vi "OP30 Verify Station.vi"(2 "Report":i32(listbox), 8 "error in (no error)":errorcluster, 11 "Ref in":T1={"MS SQL Connection"=refnum, "UDL File"=path "", "Time"="", "DCODE"="", "WIP+1"=0, "MC No?"=0, "POKAYOKE?"=FALSE, "Expected Result"="", "Result [Status]"="", "Clock"=0.0, "RFID"="", "WIP Queue"=refnum, "TS Parameter"={"ProfitCenterCode"="", "LineCode"="", "WorkOrderNumber"="", "Model"="", "Model_with_Prefix"="", "VendorCode"="", "SetParameterDateCode"="", "PokaYoke"=0, "Target"=1, "Live_DateCode"="", "CustomerPartNumber"="", "Hand"="", "sBarcode"=FALSE, "FCA"=0, "Ent_Stamp"=timestamp(0 s since 1904-01-01), "STS_CD"=0.0}, "Data_Queue"=[], "RFID Serial No."=""} {"TS Parameter"."FCA" format="%01d"; "TS Parameter"."Target" min=1 max=100000; "TS Parameter"."PokaYoke" min=0 max=1}) -> (0 "error out":errorcluster, 1 "subarray":string[](array[string]), 3 "Ref in 2":T1={"MS SQL Connection"=refnum, "UDL File"=path "", "Time"="", "DCODE"="", "WIP+1"=0, "MC No?"=0, "POKAYOKE?"=FALSE, "Expected Result"="", "Result [Status]"="", "Clock"=0.0, "RFID"="", "WIP Queue"=refnum, "TS Parameter"={"ProfitCenterCode"="", "LineCode"="", "WorkOrderNumber"="", "Model"="", "Model_with_Prefix"="", "VendorCode"="", "SetParameterDateCode"="", "PokaYoke"=0, "Target"=1, "Live_DateCode"="", "CustomerPartNumber"="", "Hand"="", "sBarcode"=FALSE, "FCA"=0, "Ent_Stamp"=timestamp(0 s since 1904-01-01), "STS_CD"=0.0}, "Data_Queue"=[], "RFID Serial No."=""} {"TS Parameter"."FCA" format="%01d"; "TS Parameter"."Target" min=1 max=100000; "TS Parameter"."PokaYoke" min=0 max=1}, 4 "Ack 2":bool)   [LabVIEW 2020]
uses:
  Controls/FV_Status.ctl
  Controls/TD SQL.ctl
  <vilib>/addons/database/Connection.llb/Conn ObjectReference.ctl
  Controls/WIP_State.ctl
  Controls/TS_Parameter.ctl
  <vilib>/Utility/miscctls.llb/LVRowAndColumnUnsignedTypeDef.ctl
  MS SQL/MS_Global.vi
  <vilib>/addons/database/_DB Variant To Data/Database Variant To Data.xnode
  <vilib>/addons/database/NI_Database_API.lvlib
panel:
  in  "Abort":bool
  out "Numeric":i32
  out "x != y?":bool
  in  "RFID_OPC":string="0029032640C1845Ag000001"
  in  "Ack":bool
  out "Over all Status":T4 caption="Data Validation"
  in  "Reason":string
  in  "RFID":string="0029032640C1845Ag000001"
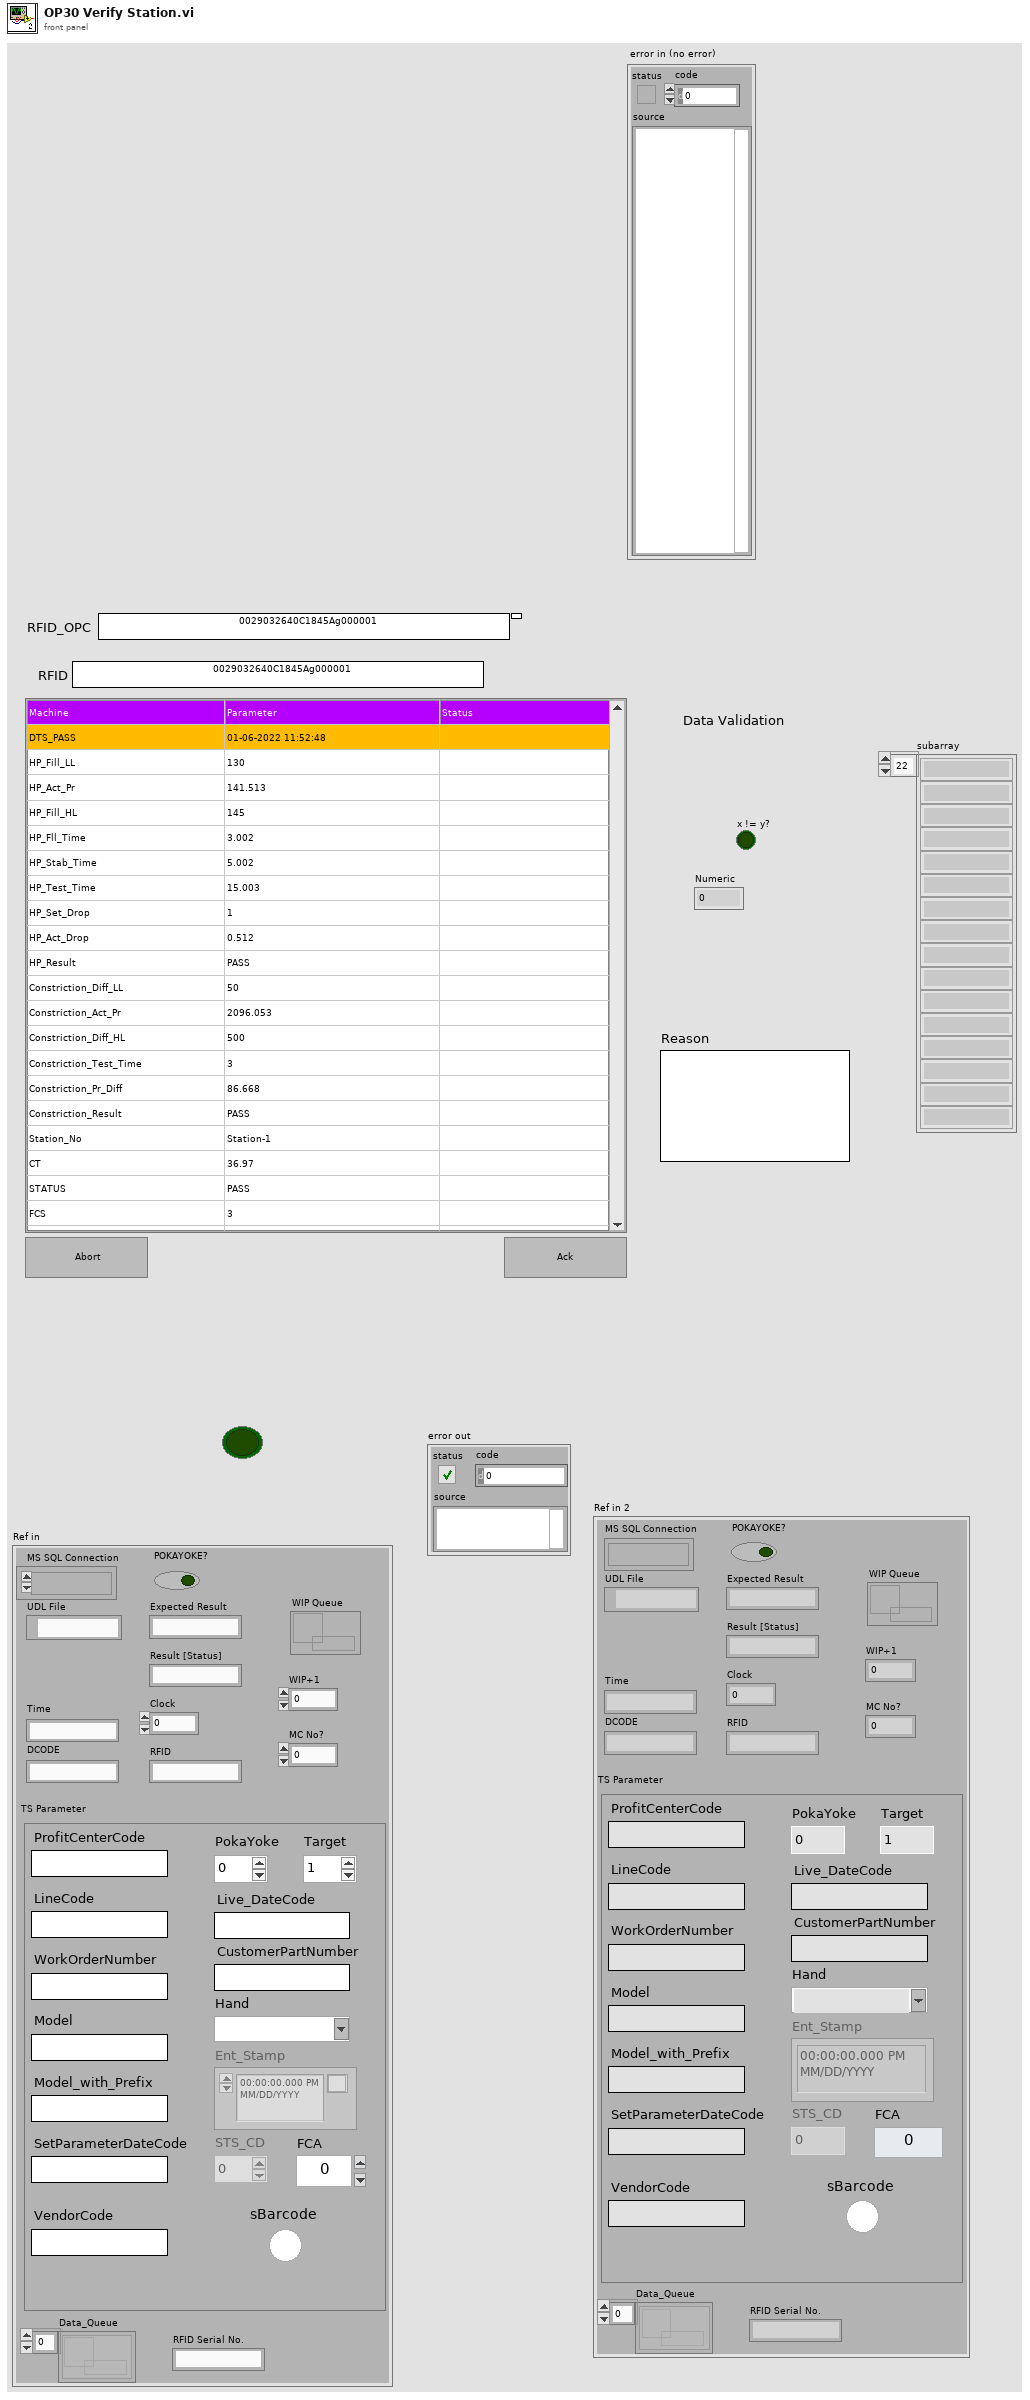
[diagram p1: front panel]
types:
  T1 = typedef "TD SQL.ctl" = cluster{"MS SQL Connection":T2, "UDL File":path, "Time":string, "DCODE":string, "WIP+1":i64, "MC No?":i32, "POKAYOKE?":bool, "Expected Result":string, "Result [Status]":string, "Clock":dbl, "RFID":string, "WIP Queue":refnum<queue>, "TS Parameter":T3, "Data_Queue":refnum<queue>[], "RFID Serial No.":string}
  T2 = typedef "NI_Database_API.lvlib/Conn ObjectReference.ctl" = refnum<k1>
  T3 = typedef "TS_Parameter.ctl" = cluster{"ProfitCenterCode":string, "LineCode":string, "WorkOrderNumber":string, "Model":string, "Model_with_Prefix":string, "VendorCode":string, "SetParameterDateCode":string, "PokaYoke":i32, "Target":i32, "Live_DateCode":string, "CustomerPartNumber":string, "Hand":string, "sBarcode":bool, "FCA":i32, "Ent_Stamp":timestamp, "STS_CD":dbl}
  T4 = typedef "FV_Status.ctl" = u16
  T5 = typedef "LVRowAndColumnUnsignedTypeDef.ctl" = cluster{"Row":u32, "Column":u32}
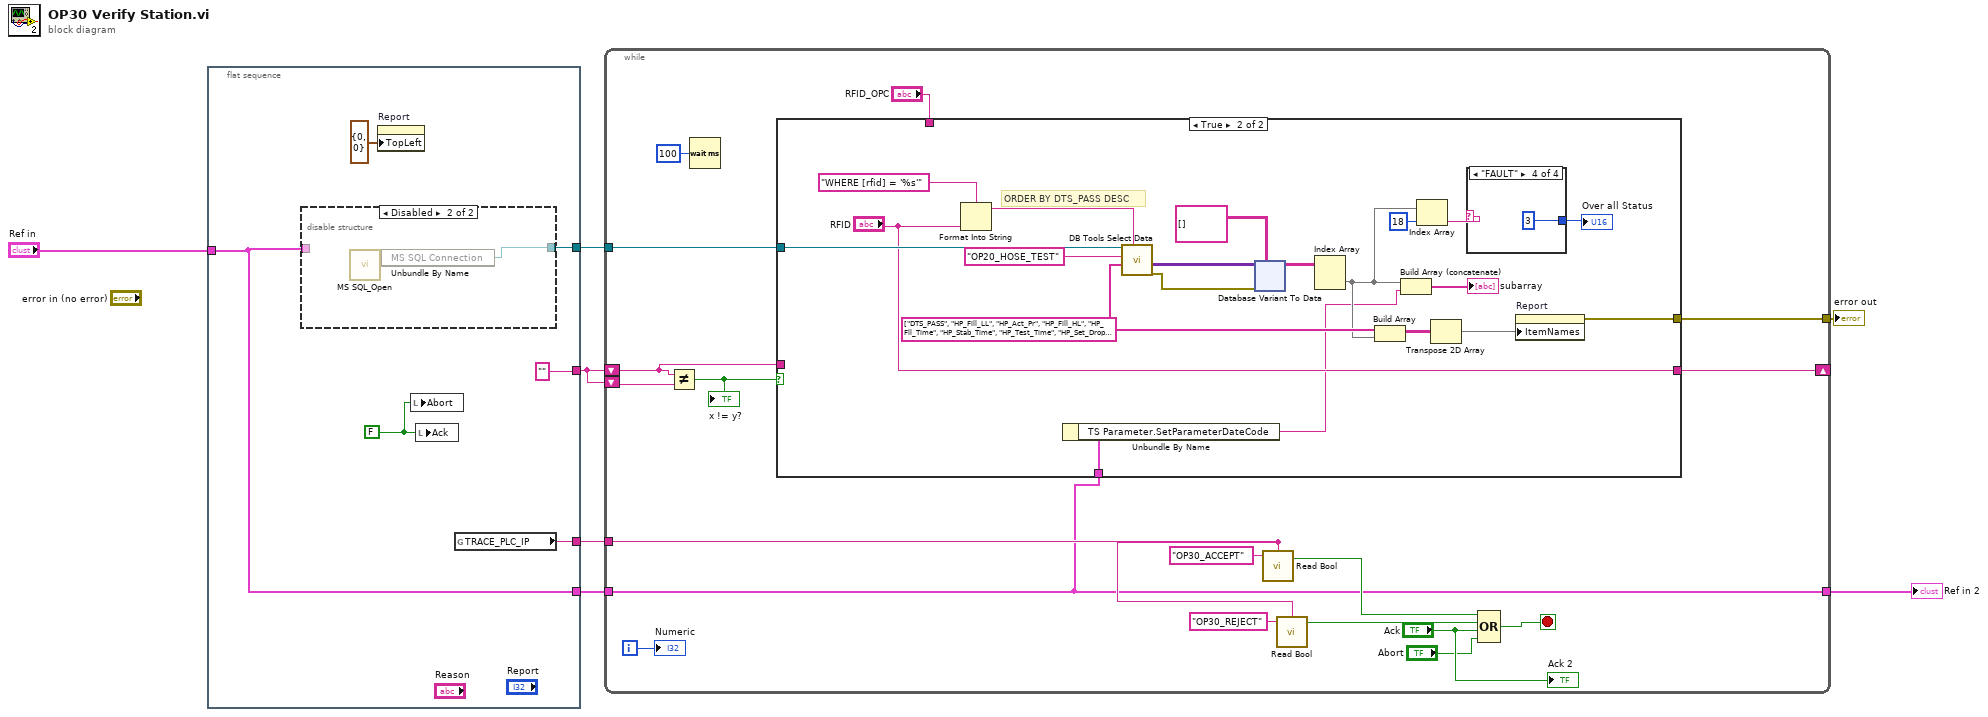
[diagram p0: block diagram]
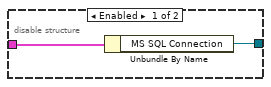
[diagram p2: hidden frame]
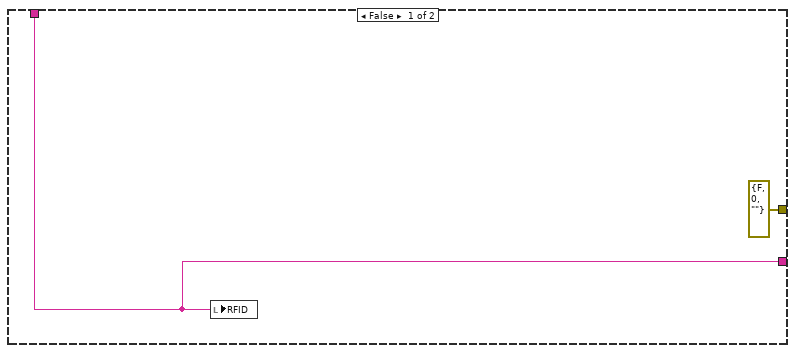
[diagram p3: hidden frame]
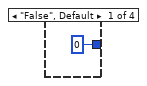
[diagram p4: hidden frame]
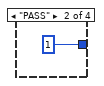
[diagram p5: hidden frame]
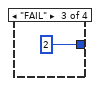
[diagram p6: hidden frame]
diagram:
  n1 = flat-sequence {
    tunnel: [w11] -> w7
    tunnel: "Ref in" -> [w12]
    tunnel: [w12] -> w4
    tunnel: ["" ("RFID")] -> w2
    tunnel: [w9] -> w1
    frame #0 {
      w8 = FALSE ("Cancel Button")
      n2 = disable-structure shown="Disabled" {
        disable-tunnel: w12 -> [w15 _]
        disable-tunnel: [w14 w16] -> w11
        frame Enabled {
          n3 = Unbundle By Name(w15) -> ("MS SQL Connection"=w14:T2)
        }
        frame Disabled {
          n4 = call "MS SQL_Open.vi"() -> ("Ref Out"=w17:T1)  [unwired: 9 in, 2 out]
          n5 = Unbundle By Name(w17) -> ("MS SQL Connection"=w16:T2)
        }
      }
      n6 = property on="Report" class="MCListbox (strict)"("TopLeft"=T5 {"Row"=0, "Column"=0} ("Top Left Visible Cell")) -> ()  [unwired: 2 in, 2 out]
      n7 = local write "Abort"(w8) -> ()
      n8 = local write "Ack"(w8) -> ()
      n9 = global read "MS_Global.vi" "TRACE_PLC_IP"() -> (w9:string)
    }
  }
  n10 = while {
    tunnel: w7 -> [w35]
    tunnel: [w34] -> w6
    tunnel: w4 -> [w18]
    tunnel: [w18] -> w3
    shift-right: [w27] -> _
    shift-left: w2 -> [w31]
    shift-left: w2 -> [w33]
    tunnel: w1 -> [w24]
    i -> [w28]
    stop <- w20 stop-if-true
    n11 = Not Equal?(x=w31, y=w33) -> (x != y?=w32:bool)
    "x != y?" <- w32
    n12 = Wait (ms)(milliseconds to wait=u32 100) -> ()  [unwired: 1 out]
    n13 = case shown="True" w32 {
      tunnel: w35 -> [_ w57]
      tunnel: [errorcluster {"status"=FALSE, "code"=0, "source"=""} ("error out") w56] -> w34
      tunnel: [w36 "RFID"] -> w27
      tunnel: w31 -> [_ _]
      tunnel: "RFID_OPC" -> [w36 _]
      tunnel: w18 -> [_ w39]
      frame False {
        n14 = local write "RFID"(w36) -> ()
      }
      frame True {
        w46 = string[] ["DTS_PASS", "HP_Fill_LL", "HP_Act_Pr", "HP_Fill_HL", "HP_Fll_Time", "HP_Stab_Time", "HP_Test_Time", "HP_Set_Drop", "HP_Act_Drop", "HP_Result", "Constriction_Diff_LL", "Constriction_Act_Pr", "Constriction_Diff_HL", "Constriction_Test_Time", "Constriction_Pr_Diff", "Constriction_Result", "Station_No", "CT", "STATUS", "FCS", "FCA", "MODELNO"] ("columns")
        # "ORDER BY DTS_PASS DESC"
        n15 = Format Into String(format string="WHERE [rfid] = '%s'" ("condition"), "RFID") -> (resulting string=w55:string)  [unwired: 2 in, 1 out]
        n16 = Unbundle By Name(w39) -> ("TS Parameter.SetParameterDateCode"=w38:string)
        n17 = call <vilib>:"DB Tools Select Data.vi"("condition"=w55, "columns"=w46, "table"="OP20_HOSE_TEST", "connection reference"=w57) -> ("error out"=w53:errorcluster, "data"=w54:variant[][])  [unwired: 2 in, 1 out]
        n18 = xnode "Database Variant To Data"("database variant"=w54, "error in (no error)"=w53, "type"=string[][] [] ("columns")) -> ("data"=w52:string[][])  [unwired: 1 out]
        n19 = Index Array(array=w52) -> (element=w41:string[])  [unwired: 2 in]
        n20 = Build Array(w46, w41) -> (w51:string[][])
        n21 = Build Array (concatenate)(w41, w38) -> (→"subarray":string[])
        n22 = Index Array(array=w41, index=18) -> (element=w49:string)
        n23 = Transpose 2D Array(2D array=w51) -> (transposed array=w50:string[][])
        n24 = case shown="\"FAULT\"" w49 {
          tunnel: [T4 0 ("Over all Status") T4 1 ("Over all Status") T4 2 ("Over all Status") T4 3 ("Over all Status")] -> w48
          frame "False", Default {
          }
          frame "PASS" {
          }
          frame "FAIL" {
          }
          frame "FAULT" {
          }
        }
        "Over all Status" <- w48
        n25 = property on="Report" class="MCListbox (strict)"("ItemNames"=w50) -> (error out=w56:errorcluster)  [unwired: 2 in, 1 out]
      }
    }
    n26 = call "Read Bool.vi"("Network Path"=w24, "Tag Name"="OP30_ACCEPT") -> ("BOOL"=w23:bool)  [unwired: 3 in]
    n27 = call "Read Bool.vi"("Network Path"=w24, "Tag Name"="OP30_REJECT") -> ("BOOL"=w22:bool)  [unwired: 3 in]
    n28 = Compound Arithmetic op=OR(w23, w22, "Ack", "Abort") -> (w20:bool)
    "Numeric" <- w28
    "Ack 2" <- "Ack"
  }
  "error out" <- w6
  "Ref in 2" <- w3
